vi "Application Launcher.vi"() -> ()   [LabVIEW 2020]
uses:
  Support/Stop User Event/Controls/User event Actions.ctl
  Support/Stop User Event/User Event - Stop.lvlib
  Support/Modules Template/Module Template.lvlib
panel:
  out "error out":errorcluster
  # "Main Launcher"
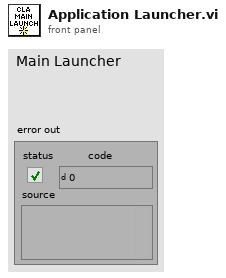
[diagram p1: front panel]
types:
  T1 = typedef "User Event - Stop.lvlib/User event Actions.ctl" = enum16{"Create", "Get Reference", "Fire Stop Event", "Destroy"}
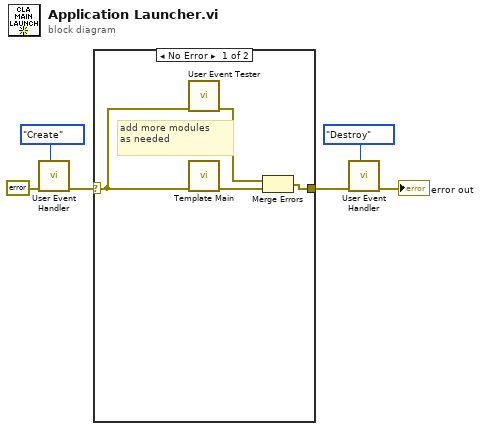
[diagram p0: block diagram]
diagram:
  n1 = call "User Event Handler.vi"("User Event Action"=User_event_Actions."Create", "error in (no error)"=errorcluster {"status"=FALSE, "code"=0, "source"=""}) -> ("error out"=w4:errorcluster)  [unwired: 8 in, 1 out]
  n2 = case shown="No Error" w4 {
    selector: w4 -> [w9 w11]
    tunnel: [w10 w11] -> w3
    frame No Error {
      # "add more modules\nas needed"
      n3 = call "User Event Tester.vi"("error in (no error)"=w9) -> ("error out"=w7:errorcluster)  [unwired: 10 in]
      n4 = call "Template Main.vi"("error in (no error)"=w9) -> ("error out"=w8:errorcluster)  [unwired: 10 in]
      n5 = Merge Errors(w7, w8) -> (w10:errorcluster)
    }
    frame Error {
    }
  }
  n6 = call "User Event Handler.vi"("User Event Action"=User_event_Actions."Destroy", "error in (no error)"=w3) -> ("error out"=→"error out":errorcluster)  [unwired: 8 in, 1 out]
